vi "setTriggering.vi"(8 "error in (no error)":errorcluster, 10 "Triggering":T1, 11 "CameraSettingsManager.lvclass in":refnum<class "CameraSettingsManager.lvclass">) -> (0 "error out":errorcluster, 3 "CameraSettingsManager.lvclass out":refnum<class "CameraSettingsManager.lvclass">)   [LabVIEW 2009, in "Tools.lvlib" / "Settings.lvlib" / "CameraSettingsManager.lvclass"]
uses:
  CameraSettingsManager.lvclass
  CameraSettingsManager.lvclass/CameraSettingsManager.ctl
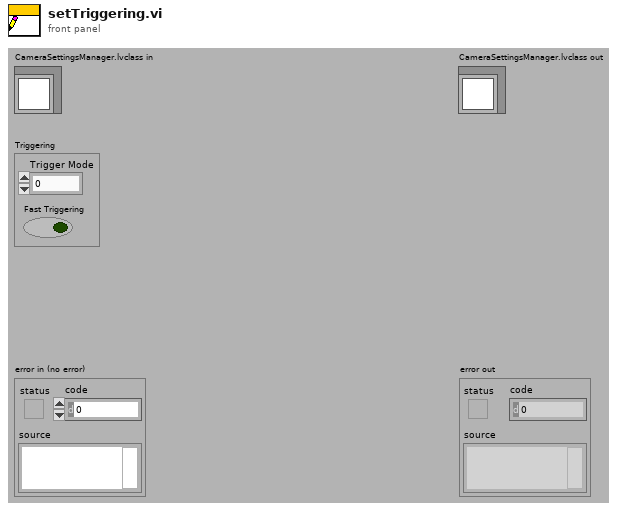
[diagram p1: front panel]
types:
  T1 = cluster{"Trigger Mode":dbl, "Fast Triggering":bool}
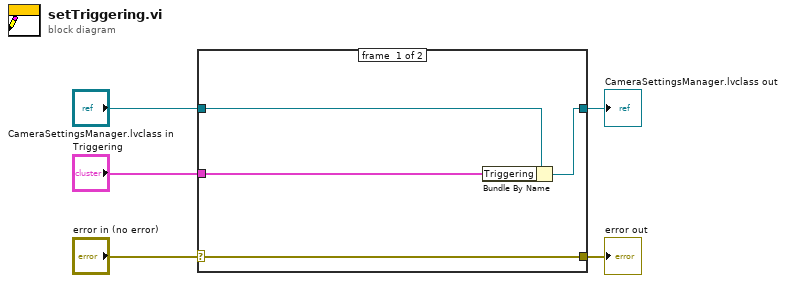
[diagram p0: block diagram]
diagram:
  n1 = case shown="No Error" "error in (no error)" {
    selector: "error in (no error)" -> [w9 w10]
    tunnel: [w9 w10] -> w4
    tunnel: [w7 w11] -> w2
    tunnel: "CameraSettingsManager.lvclass in" -> [w8 w11]
    tunnel: "Triggering" -> [w6 _]
    frame #0 {
      n2 = Bundle By Name(cluster=w8, "Triggering"=w6) -> (w7:refnum<class "CameraSettingsManager.lvclass">)
    }
    frame #1 {
    }
  }
  "error out" <- w4
  "CameraSettingsManager.lvclass out" <- w2
